vi "alex_initialize_sub_vi.vi"(0 "VISA Refnum in":refnum<visa-resource-name>, 1 "Bytes to read (100)":u32=100, 2 "Wait before read (0ms)":u32, 5 "Serial Link (RS232)":enum16{"RS232", "USB"}(ring), 7 "error in (no error) 2":errorcluster, 9 "error in (no error)":errorcluster, 11 "error in (no error)":errorcluster, 12 "ID Query (True)":bool=TRUE, 13 "Reset (False)":bool) -> (4 "Returned string":string, 6 "error out 2":errorcluster={"status"=TRUE, "code"=-1073807339, "source"="VISA Read dans Newport ESP301.lvlib:Write Command and Read.vi"}, 8 "error out 3":errorcluster, 15 "error out":errorcluster {"code" format="%.0x"})   [LabVIEW 2017]
uses:
  Newport ESP301/Newport ESP301.lvlib
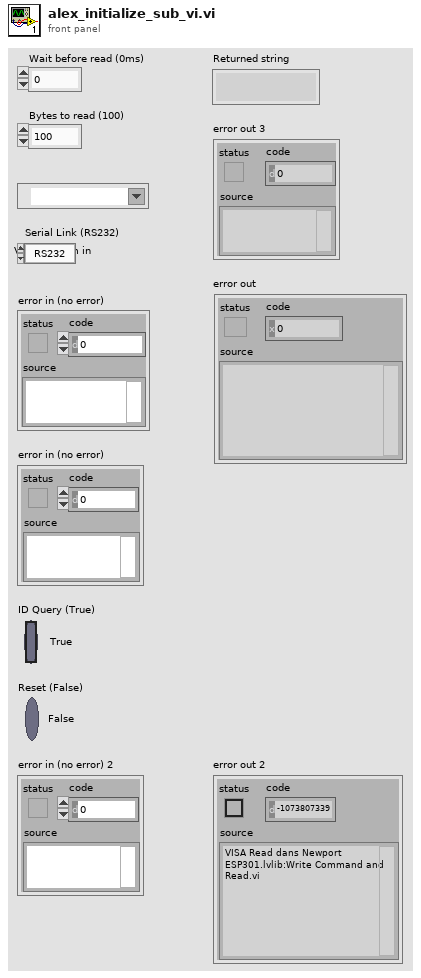
[diagram p1: front panel]
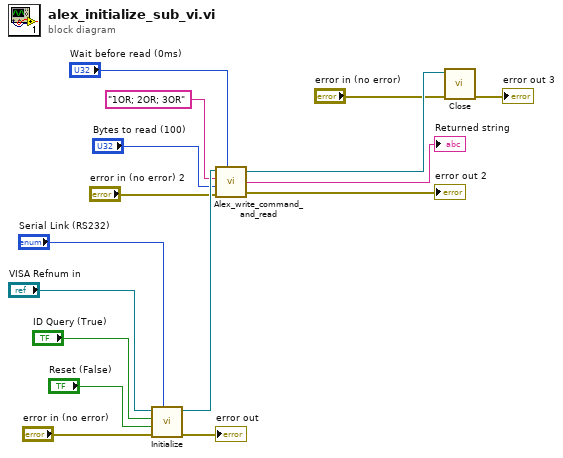
[diagram p0: block diagram]
diagram:
  n1 = call "Initialize.vi"("VISA resource name"="VISA Refnum in", "ID Query (True)"="ID Query (True)", "Reset (False)"="Reset (False)", "error in (no error)"="error in (no error)", "Serial Link (RS232)"="Serial Link (RS232)") -> ("VISA resource name out"=w13:refnum<visa-resource-name>, "error out"=→"error out":errorcluster)  [unwired: 4 in]
  n2 = call "Alex_write_command_and_read.vi"("VISA resource name"=w13, "Wait before read (0ms)"="Wait before read (0ms)", "Command"="1OR; 2OR; 3OR", "Bytes to read (100)"="Bytes to read (100)", "error in (no error)"="error in (no error) 2") -> ("VISA resource name out"=w16:refnum<visa-resource-name>, "Returned string"=→"Returned string":string, "error out"=→"error out 2":errorcluster)  [unwired: 1 in]
  n3 = call "Close.vi"("error in (no error)"="error in (no error)", "VISA resource name"=w16) -> ("error out"=→"error out 3":errorcluster)  [unwired: 9 in]
